vi "Data Read.vi"(7 "Retry Attempts (0)":i32 min=0, 8 "error in (no error)":errorcluster, 10 "Bytes to read (1024)":u32=1024, 11 "VISA Refnum in":refnum<visa-resource-name>) -> (0 "error out":errorcluster, 2 "Response Cluster":T1 {"Command ID" format="%x"}, 3 "VISA Refnum out":refnum<visa-resource-name>, 5 "read buffer (debug)":string)   [LabVIEW 2020, in "Omega Platinum Series.lvlib"]
uses:
  Omega Platinum Series.lvlib
  Type Defs/Response.ctl
  <vilib>/Utility/sysdir.llb/System Directory Type.ctl
panel:
  out "Retries":i32
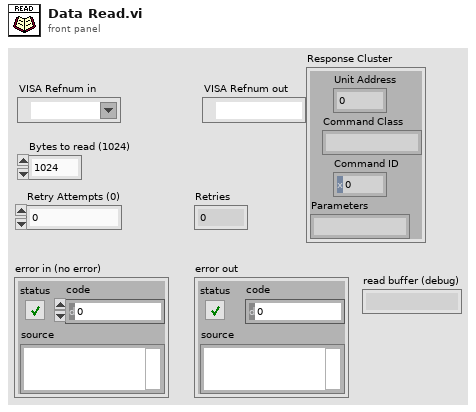
[diagram p1: front panel]
types:
  T1 = typedef "Omega Platinum Series.lvlib/Response.ctl" = cluster{"Unit Address":i32, "Command Class":string, "Command ID":u32, "Parameters":string}
  T2 = typedef "System Directory Type.ctl" = i32
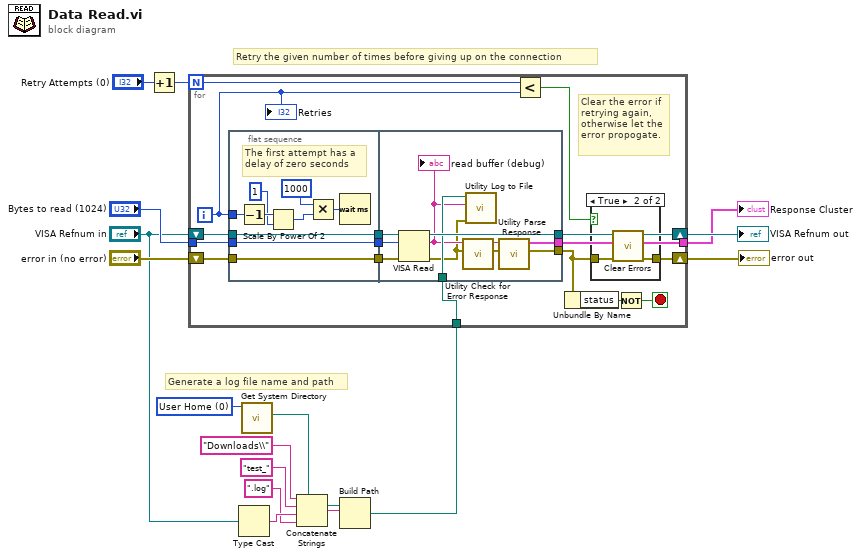
[diagram p0: block diagram]
diagram:
  w7 = T2 0 items=["User Home"=0, "User Desktop"=1, "User Documents"=2, "User Application Data"=3, "User Preferences"=4, "User Temporary"=5, "Public Documents"=6, "Public Application Data"=7, "Public Preferences"=8, "Public Cache"=13, "System Core Libraries"=9, "System Installed Libraries"=10, "Application Files"=11, "Boot Volume Root"=12] ("system directory type")
  # "Retry the given number of times before giving up on the connection"
  # "Generate a log file name and path"
  n1 = Increment(x="Retry Attempts (0)") -> (x+1=w1:i32)
  n2 = Type Cast(x="VISA Refnum in") -> (*(type *) &x=w11:string)  [unwired: 1 in]
  n3 = call <vilib>:"Get System Directory.vi"("system directory type"=w7) -> ("system directory"=w8:path)  [unwired: 10 in]
  n4 = Concatenate Strings("Downloads\\", "test_", w11, ".log") -> (w10:string)
  n5 = Build Path(base path=w8, name or relative path=w10) -> (appended path=w3:path)
  n6 = for {
    N: w1 -> [w17]
    tunnel: "Bytes to read (1024)" -> [w31]
    tunnel: [w27] -> w13
    tunnel: w3 -> [w28]
    shift-right: [w20] -> w4
    shift-left: "error in (no error)" -> [w30]
    shift-right: [w32] -> w16
    shift-left: "VISA Refnum in" -> [w29]
    i -> [w18]
    stop <- w21 stop-if-true
    # "Clear the error if\nretrying again,\notherwise let the\nerror propogate."
    n7 = flat-sequence {
      tunnel: w29 -> [w42]
      tunnel: w30 -> [w43]
      tunnel: w31 -> [w44]
      tunnel: [w44] -> w26
      tunnel: [w43] -> w25
      tunnel: [w42] -> w24
      tunnel: w18 -> [w36]
      tunnel: [w55] -> w32
      tunnel: [w46] -> w23
      tunnel: w28 -> [w51]
      tunnel: [w45] -> w27
      tunnel: w26 -> [w54]
      tunnel: w25 -> [w53]
      tunnel: w24 -> [w52]
      frame #0 {
        # "The first attempt has a \ndelay of zero seconds"
        n8 = Decrement(x=w36) -> (x-1=w38:i32)
        n9 = Scale By Power Of 2(n=w38, x=1) -> (x*2^n=w41:i32)
        n10 = Multiply(x=1000, y=w41) -> (x*y=w39:i32)
        n11 = Wait (ms)(milliseconds to wait=w39) -> ()  [unwired: 1 out]
      }
      frame #1 {
        n12 = VISA Read(VISA resource name=w52, byte count=w54, error in (no error)=w53) -> (VISA resource name out=w55:refnum<visa-resource-name>, read buffer=w50:string, error out=w48:errorcluster)  [unwired: 1 out]
        "read buffer (debug)" <- w50
        n13 = call "Utility Check for Error Response.vi"("error in (no error)"=w48, "Response String (in)"=w50) -> ("error out"=w47:errorcluster, "Response String (out)"=w49:string)  [unwired: 8 in]
        n14 = call "Utility Log to File.vi"("error in (no error)"=w48, "Command"=w50, "Log File Path"=w51) -> ()  [unwired: 8 in, 1 out]
        n15 = call "Utility Parse Response.vi"("error in (no error)"=w47, "Response String"=w49) -> ("error out"=w46:errorcluster, "Response Cluster"=w45:T1)  [unwired: 8 in]
      }
    }
    n16 = Less?(x=w17, y=w18) -> (x < y?=w19:bool)
    n17 = Unbundle By Name(w23) -> ("status"=w22:bool)
    n18 = case shown="True" w19 {
      tunnel: w23 -> [w33 w35]
      tunnel: [w33 w34] -> w20
      frame False {
      }
      frame True {
        n19 = call <vilib>:"Clear Errors.vi"("error in (no error)"=w35) -> ("error out"=w34:errorcluster)  [unwired: 5 in, 1 out]
      }
    }
    n20 = Not(x=w22) -> (.not. x?=w21:bool)
    "Retries" <- w18
  }
  "VISA Refnum out" <- w16
  "error out" <- w4
  "Response Cluster" <- w13
